vi "DataPtNDateWrite2File 4.vi"(6 "Calling VIs path":path, 7 "Save the Graph":bool, 8 "Comments to go in Header":string, 9 "Graph to be Saved":cluster{"Time":dbl[], "Peak-bkg Value":dbl[]}(graph), 10 "ProjectName":string="PrExpt", 11 "Folder path input":path=path "C:/Users/Lab/Desktop/Data/Wavemeter") -> (1 "Column Names":string[](array[string])=["Xname", "Yname"], 2 "Header":string, 3 "new file path that was created":path)   [LabVIEW 2016]
doc: "This takes a graph as input and writes it to a file. It grabs the column labels from the graph display.\nThe file naming is automated with DataFileCreator.vi\nDataFileCreator.vi is given an input Folder path and ProjectName this VI creates the next data file in the format \n2017-09-17ProjectName#001\nIt only checks the latest file in the folder to decide if \na sequence with today's date already exists.\nIf the file sequence has not been started, it creates one begining with #001\nIf it happens that it tries to create a file that already exists, a dialog pops up\nasking for a new name.\nAdd any comments you want saved in the file.\nPush the \"Save the Graph\" if you want the save to happen. This eliminates the need for the query in the main program."
uses:
  <vilib>/Utility/file.llb/Write To Spreadsheet File (DBL).vi
panel:
  in  "DataPt2BStored":dbl
  # "This takes a graph as input and writes it to a file. It grabs the column labels from the graph display.\nThe file naming is automated with DataFileCreator.vi\nDataFileCreator.vi is given an input Folder path and ProjectName this VI creates the next data file in the format \n2017-09-17ProjectName#001\nIt only checks the latest file in the folder to decide if \na sequence with today's date already exists.\nIf the file sequence has not been started, it creates one begining with #001\nIf it happens that it tries to create a file that already exists, a dialog pops up\nasking for a new name.\nAdd any comments you want saved in the file.\nPush the \"Save the Graph\" if you want the save to happen. This eliminates the need for the query in the main program."
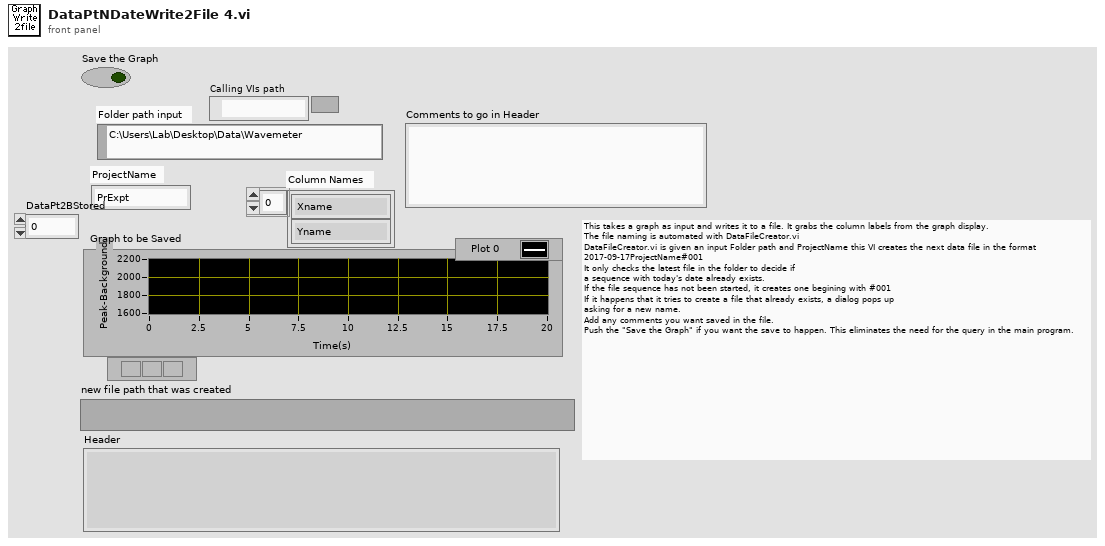
[diagram p1: front panel]
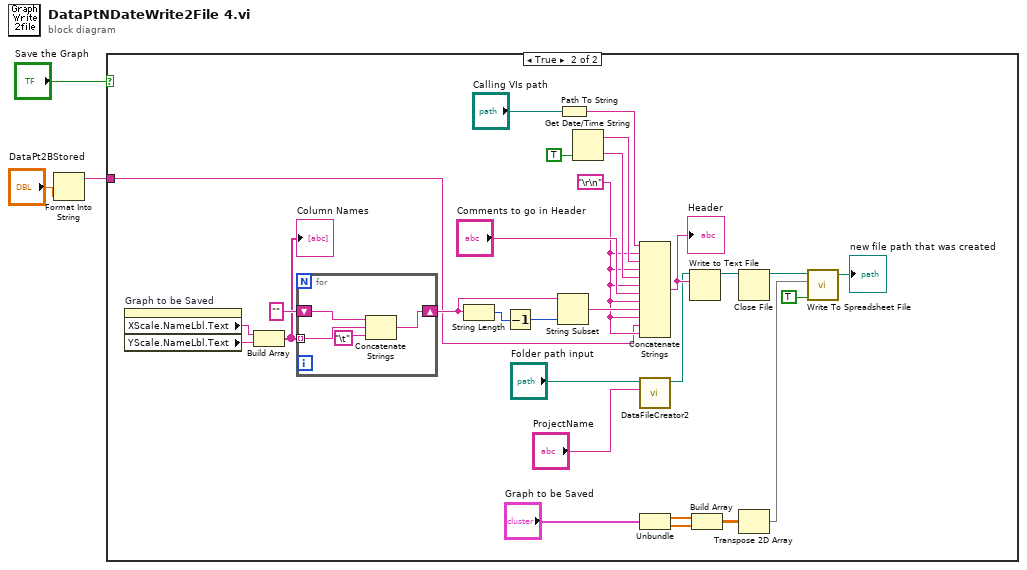
[diagram p0: block diagram]
diagram:
  n1 = Format Into String("DataPt2BStored") -> (resulting string=w1:string)  [unwired: 3 in, 1 out]
  n2 = case shown="True" "Save the Graph" {
    tunnel: w1 -> [_ w4]
    frame False {
    }
    frame True {
      w5 = "\r\n"
      n3 = property on="Graph to be Saved" class="XYGraph (strict)"() -> ("XScale.NameLbl.Text"=w9:string, "YScale.NameLbl.Text"=w8:string)  [unwired: 2 in, 2 out]
      n4 = Build Array(w9, w8) -> (w7:string[])
      "Column Names" <- w7
      n5 = for {
        shift-right: [w35] -> w26
        shift-left: "" -> [w36]
        tunnel: w7 -> [w33] mode=indexing
        n6 = Concatenate Strings(w36, w33, "\t") -> (w35:string)
      }
      n7 = String Length(string=w26) -> (length=w25:i32)
      n8 = Decrement(x=w25) -> (x-1=w24:i32)
      n9 = String Subset(string=w26, length (rest)=w24) -> (substring=w14:string)  [unwired: 1 in]
      n10 = Path To String(path="Calling VIs path") -> (string=w31:string)
      n11 = Get Date/Time String(want seconds? (F)=TRUE) -> (date string=w30:string, time string=w29:string)  [unwired: 2 in]
      n12 = Concatenate Strings(w31, w5, w30, w5, w29, w5, "Comments to go in Header", w5, w14, w5, w4, w5) -> (w28:string)
      "Header" <- w28
      n13 = call "DataFileCreator2.vi"("ProjectName"="ProjectName", "Folder path input"="Folder path input") -> ("NewFilePath"=w18:path)  [unwired: 8 in, 1 out]
      n14 = Unbundle("Graph to be Saved") -> ("Time"=w11:dbl[], "Peak-bkg Value"=w10:dbl[])
      n15 = Write to Text File(file (use dialog)=w18, text=w28) -> (refnum out=w17:refnum<file>)  [unwired: 2 in, 2 out]
      n16 = Build Array(w11, w10) -> (w32:dbl[][])
      n17 = Close File(refnum=w17) -> (path=w16:path)  [unwired: 1 in, 1 out]
      n18 = Transpose 2D Array(2D array=w32) -> (transposed array=w27:dbl[][])
      n19 = call-poly <vilib>:"Write To Spreadsheet File.vi"("append to file? (new file:F)"=TRUE, "2D data"=w27, "file path (dialog if empty)"=w16) -> ("new file path (Not A Path if cancelled)"=→"new file path that was created":path)  [unwired: 5 in]
    }
  }
